vi "VdTcpIP_Delete.vi"(0 "reference in":refnum<class "VdTcpIP.lvclass">, 2 "Force delete":bool, 5 "error in (no error)":errorcluster) -> (14 "reference out":refnum<class "VdTcpIP.lvclass">, 15 "# of objects":i32, 19 "error out":errorcluster)   [LabVIEW 2020, in "VdTcpIP.lvclass"]
doc: "Deletes a VdSocket object created with the VdSocket new VI and returns the contents of the object.\n\n[GOOP 2.0.11]"
uses:
  <instrlib>/_InstrumentDrivers/VdCommunication/VdTcpIP_class/VdTcpIP.lvclass
  <instrlib>/_InstrumentDrivers/VdCommunication/VdTcpIP_class/VdTcpIP.lvclass/VdTcpIP.ctl
  <vilib>/addons/_goop3.llb/3GOOPStates.ctl
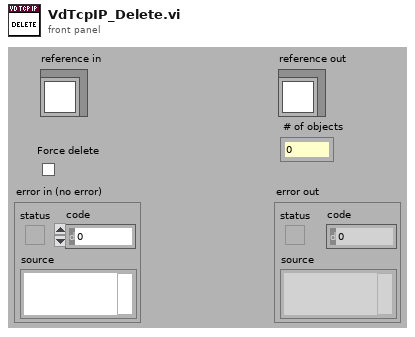
[diagram p1: front panel]
types:
  T1 = typedef "3GOOPStates.ctl" = enum16{"Set", "Get", "New", "Delete", "Clear", "Test and get", "Unlock data", "Information", "Look up existing", "New or look up existing", "Test and get shared", "Get shared", "Set shared", "Unlock shared", "Find dynamic method", "Register dynamic method", "Preload dynamic method", "Probe", "Cast to more generic", "Cast to more specific"}
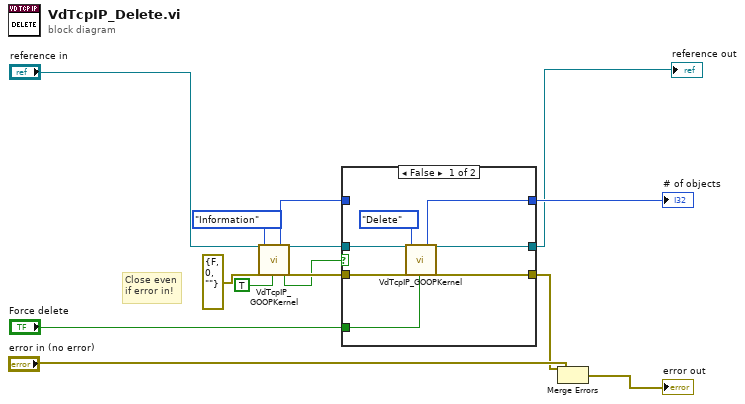
[diagram p0: block diagram]
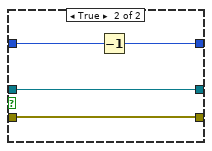
[diagram p2: hidden frame]
diagram:
  # "Close even\nif error in!"
  n1 = call <instrlib>:"VdTcpIP_GOOPKernel.vi"("Ref in"="reference in", "error in (no error)"=errorcluster {"status"=FALSE, "code"=0, "source"=""}, "Action"=3GOOPStates."Information", "Misc"=TRUE ("First try?")) -> ("# of objects"=w7:i32, "IsSubclass?"=w2:bool, "Ref out"=w10:refnum<class "VdTcpIP.lvclass">, "error out"=w9:errorcluster)  [unwired: 13 in, 7 out]
  n2 = case shown="False" w2 {
    tunnel: w10 -> [w21 w22]
    tunnel: [w20 w23] -> w12
    tunnel: [w18 w25] -> w11
    tunnel: w9 -> [w19 w23]
    tunnel: w7 -> [_ w24]
    tunnel: [w16 w22] -> w3
    tunnel: "Force delete" -> [w15 _]
    frame False {
      n3 = call <instrlib>:"VdTcpIP_GOOPKernel.vi"("Ref in"=w21, "error in (no error)"=w19, "Action"=3GOOPStates."Delete", "Misc"=w15) -> ("# of objects"=w18:i32, "Ref out"=w16:refnum<class "VdTcpIP.lvclass">, "error out"=w20:errorcluster)  [unwired: 13 in, 8 out]
    }
    frame True {
      n4 = Decrement(x=w24) -> (x-1=w25:i32)
    }
  }
  "# of objects" <- w11
  "reference out" <- w3
  n5 = Merge Errors("error in (no error)", w12) -> (→"error out":errorcluster)
